vi "Global Y.vi"() -> ()   [LabVIEW 2015]
panel:
  in  "Y":dbl
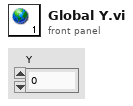
[diagram p1: front panel]
diagram:
